vi "Filter Test.vi"() -> ()   [LabVIEW 2020, in "Tests.lvlib"]
uses:
  Tests.lvlib
  3f45bdbf-d47b-438a-9a5f-3f6d8b831ff2.vi
  String Predicate.vi
panel:
  out "Filtered Array 2":string[](array[string])
  out "Filtered Array":dbl[](array[numeric])
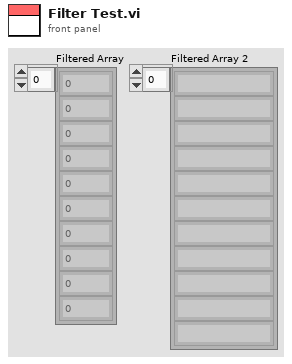
[diagram p1: front panel]
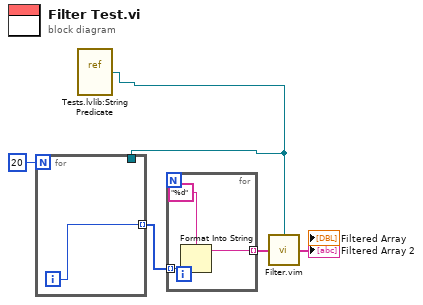
[diagram p0: block diagram]
diagram:
  n1 = vi-ref "Tests.lvlib:String Predicate.vi"() -> (w2:refnum<vi>)
  n2 = for {
    N: 20 -> [_]
    tunnel: [w6] -> w4 mode=indexing
    tunnel: w2 -> [_]
    i -> [w6]
  }
  n3 = for {
    tunnel: w4 -> [w8] mode=indexing
    tunnel: [w7] -> w3 mode=indexing
    n4 = Format Into String(format string="%d", w8) -> (resulting string=w7:string)  [unwired: 2 in, 1 out]
  }
  n5 = call "Filter.vim"("Predicate"=w2, "Array"=w3) -> ("Filtered Array"=→"Filtered Array 2":string[])  [unwired: 2 in]
